vi "ManageRefs_FGV.vi"(7 "ManRef_mods":T1, 8 "error in":errorcluster, 11 "DataIn":variant) -> (0 "error out":errorcluster, 3 "DataOut":variant)   [LabVIEW 2017]
uses:
  ManRef_mods.ctl
  ManRef_AsterData.ctl
  ManRef_ShootData.ctl
  Asteroid/Asteroid_data.ctl
  GameConfig/GameConfig_data.ctl
  Asteroid/Asteroid_states.ctl
  Spaceship/Shoot/Shoot_states.ctl
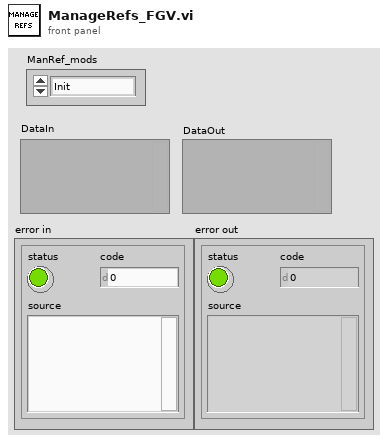
[diagram p1: front panel]
types:
  T1 = typedef "ManRef_mods.ctl" = enum16{"Init", "NewAster", "MoveAll", "DestroyAster", "NewShoot", "DestroyShot", "CheckColision", "End"}
  T2 = typedef "ManRef_ShootData.ctl" = cluster{"ID":i32, "ShootObjectRef":refnum<vi>}
  T3 = typedef "ManRef_AsterData.ctl" = cluster{"ID":i32, "AsterObjectRef":refnum<vi>}
  T4 = typedef "Asteroid_data.ctl" = cluster{"Veloc":dbl, "Direction":dbl, "Size":i32, "displayRef":refnum<vi>, "Max X":dbl, "Max Y":dbl, "Xpos":dbl, "Ypos":dbl, "ID":i32, "Config":T5}
  T5 = typedef "GameConfig_data.ctl" = cluster{"SpaceShip":cluster{"Angle":dbl, "SideLenght":dbl, "MaxLinearVeloc":dbl, "MaxAngularVeloc":dbl, "LinearAceleration":dbl, "AngularAceleration":dbl}, "Physics":cluster{"LinearDragFactor":dbl, "AngularDragFactor":dbl}, "Asteroids":cluster{"MaxSize":dbl, "MaxDivisions":i32, "MaxVeloc":dbl, "MinVeloc":dbl, "Fill":bool}, "Environment":cluster{"MaxAsteroids":i32, "TimeIncrement":dbl, "AsterProbCreation":dbl, "LogEnabled":bool}, "Shots":cluster{"MinTimeShots":dbl, "ShotSize":dbl, "ShotSpeed":dbl}}
  T6 = typedef "Shoot_states.ctl" = enum16{"Init", "Move", "Draw", "Destroy"}
  T7 = typedef "Asteroid_states.ctl" = enum16{"Init", "Move", "Split", "Draw", "Destroy"}
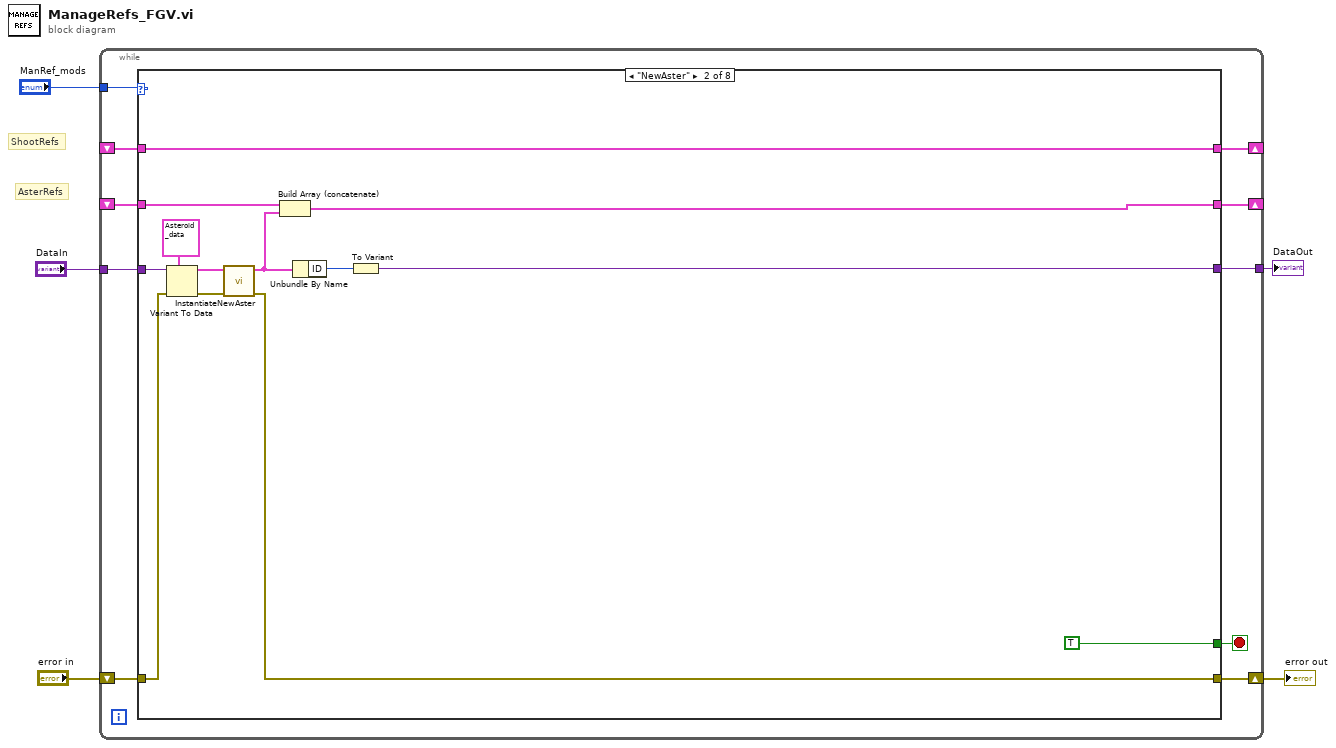
[diagram p0: block diagram]
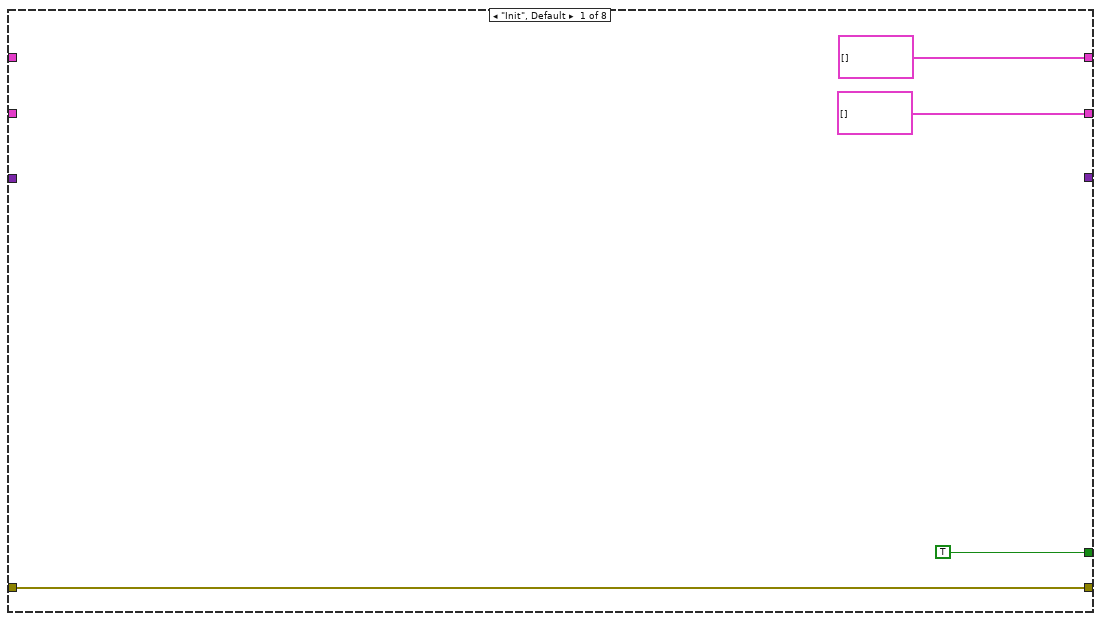
[diagram p2: hidden frame]
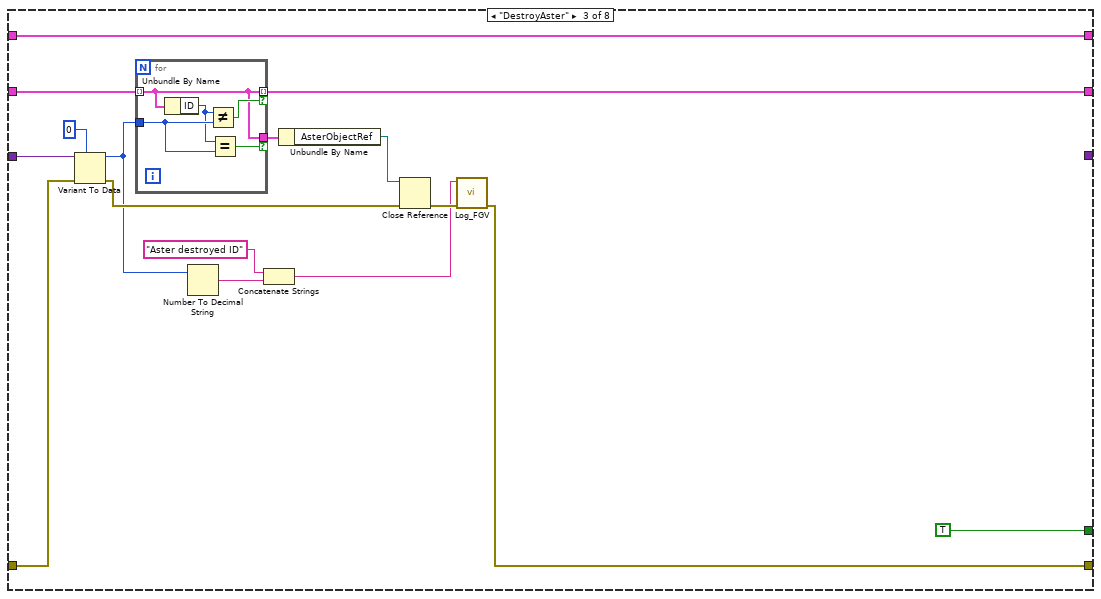
[diagram p3: hidden frame]
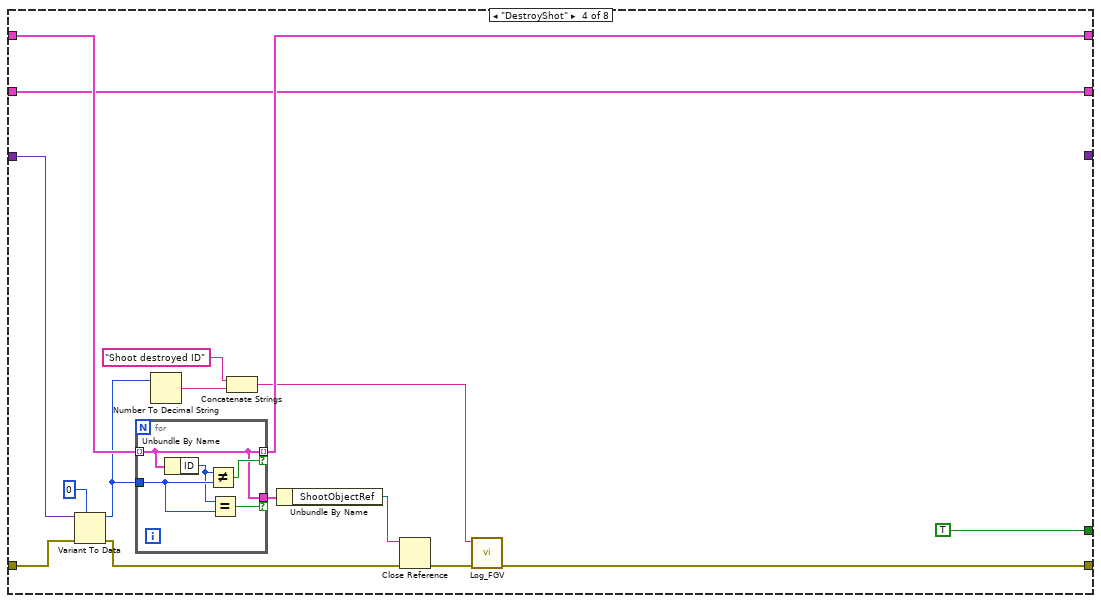
[diagram p4: hidden frame]
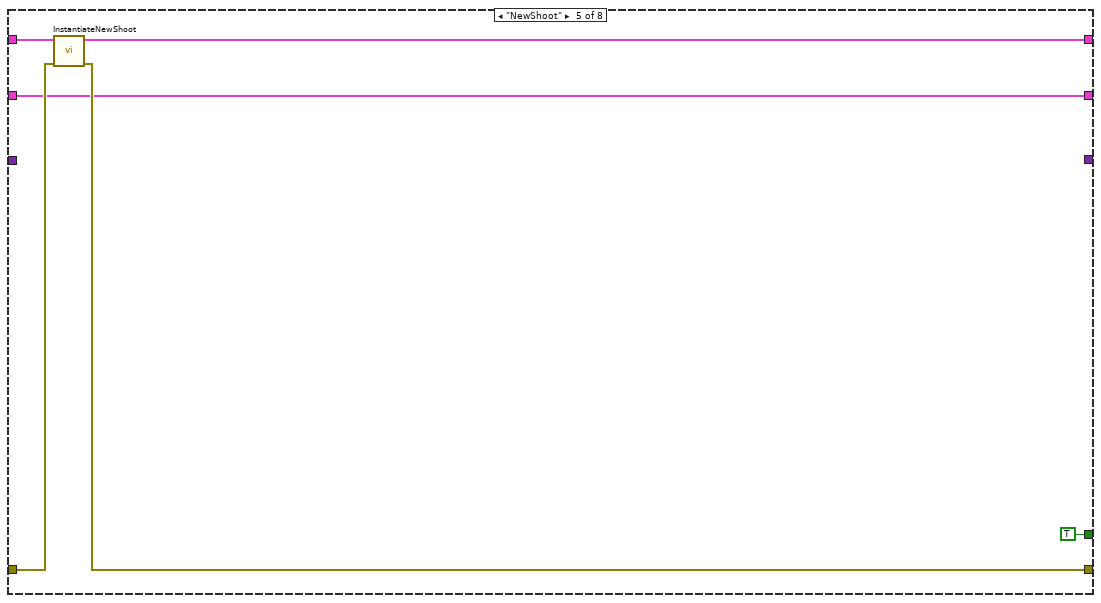
[diagram p5: hidden frame]
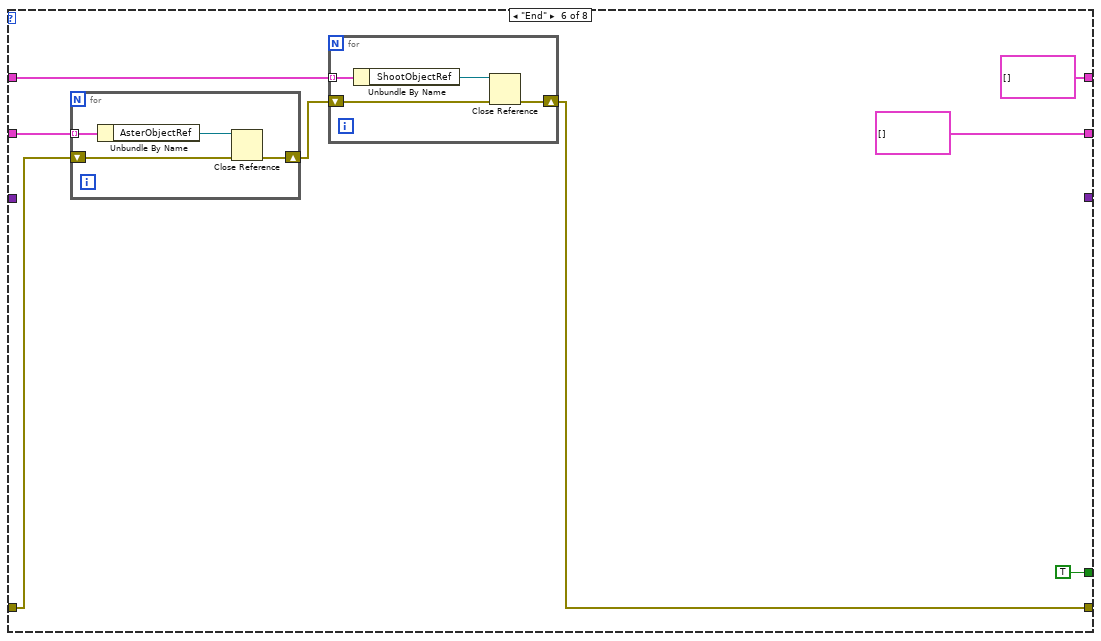
[diagram p6: hidden frame]
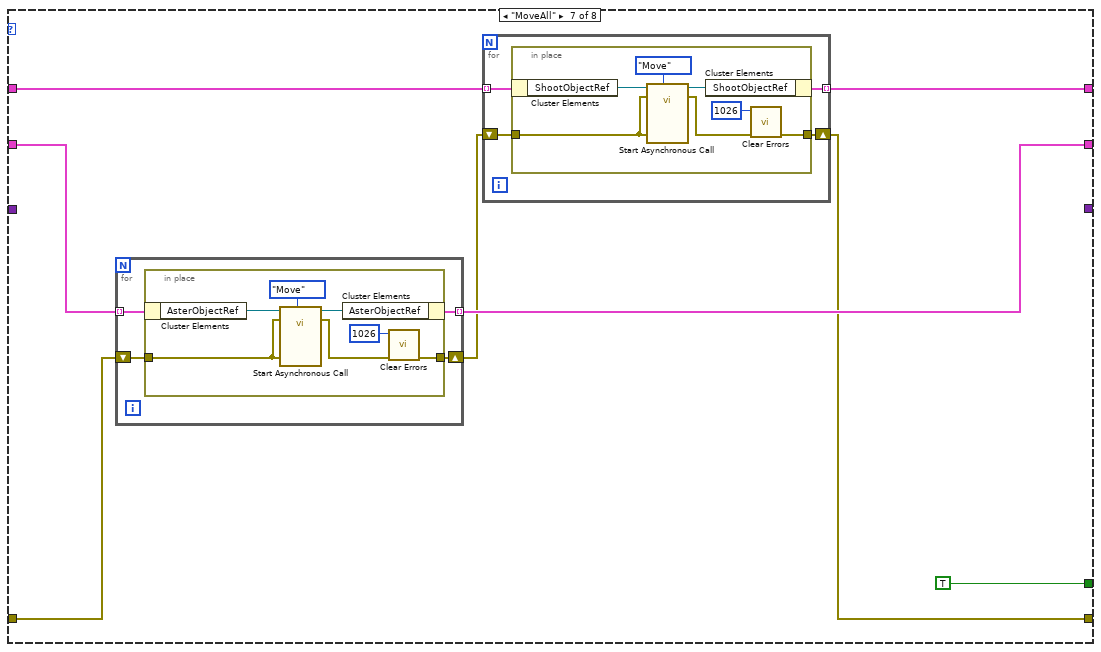
[diagram p7: hidden frame]
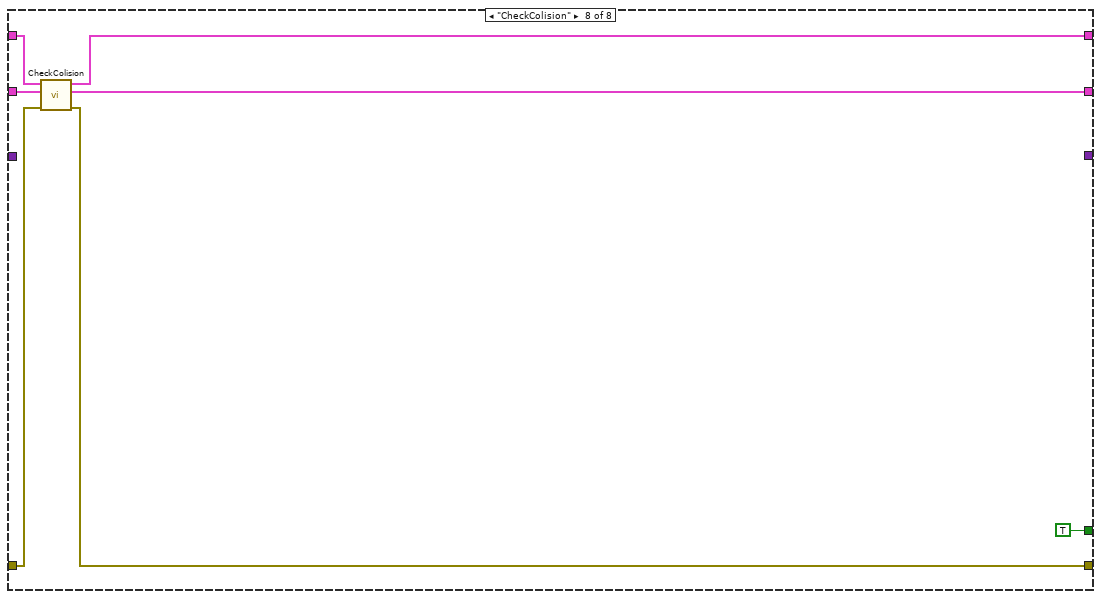
[diagram p8: hidden frame]
diagram:
  # "AsterRefs"
  # "ShootRefs"
  n1 = while {
    shift-right: [w12] -> w4
    shift-left: "error in" -> [w15]
    tunnel: "DataIn" -> [w14]
    tunnel: "ManRef_mods" -> [w13]
    shift-right: [w11] -> _
    shift-left: _ -> [w10]
    shift-right: [w8] -> _
    shift-left: _ -> [w7]
    tunnel: [w6] -> w1
    stop <- w9 stop-if-true
    n2 = case shown="\"NewAster\"" w13 {
      tunnel: w15 -> [w19 w24 w47 w68 w80 w86 w103 w132]
      tunnel: w14 -> [_ w32 w48 w69 _ _ _ _]
      tunnel: [w19 w29 w33 w54 w78 w82 w97 w127] -> w12
      tunnel: [T3[] [] ("appended array") w27 w44 w60 w75 T3[] [] ("appended array") w102 w131] -> w11
      tunnel: w10 -> [_ w28 w45 w60 w75 w87 w104 w133]
      tunnel: [TRUE ("empty?") TRUE ("empty?") TRUE ("empty?") TRUE ("empty?") TRUE ("empty?") TRUE ("empty?") TRUE ("empty?") TRUE ("empty?")] -> w9
      tunnel: [T2[] [] ("Array") w25 w39 w61 w76 T2[] [] ("Array") w98 w128] -> w8
      tunnel: w7 -> [_ w25 w39 w62 w77 w84 w100 w129]
      tunnel: [_ w20 _ _ _ _ _ _] -> w6
      frame "Init", Default {
      }
      frame "NewAster" {
        n3 = Variant To Data(error in=w24, type=T4 {"Veloc"=0.0, "Direction"=0.0, "Size"=0, "displayRef"=refnum, "Max X"=0.0, "Max Y"=0.0, "Xpos"=0.0, "Ypos"=0.0, "ID"=0, "Config"={"SpaceShip"={"Angle"=30.0, "SideLenght"=2.0, "MaxLinearVeloc"=10.0, "MaxAngularVeloc"=10.0, "LinearAceleration"=1.0, "AngularAceleration"=1.0}, "Physics"={"LinearDragFactor"=1.0, "AngularDragFactor"=1.0}, "Asteroids"={"MaxSize"=6.0, "MaxDivisions"=3, "MaxVeloc"=8.0, "MinVeloc"=1.0, "Fill"=FALSE}, "Environment"={"MaxAsteroids"=10, "TimeIncrement"=0.1, "AsterProbCreation"=0.1, "LogEnabled"=FALSE}, "Shots"={"MinTimeShots"=10.0, "ShotSize"=0.1, "ShotSpeed"=0.1}}} ("AsteroidData"), Variant=w32) -> (data=w30:T4, error out=w23:errorcluster)
        n4 = call "InstantiateNewAster.vi"("error in"=w23, "BaseAsteroidData"=w30) -> ("error out"=w29:errorcluster, "AsterRef"=w22:T3)  [unwired: 8 in]
        n5 = Build Array (concatenate)(w28, w22) -> (w27:T3[])
        n6 = Unbundle By Name(w22) -> ("ID"=w21:i32)
        n7 = To Variant(anything=w21) -> (Variant=w20:variant)
      }
      frame "DestroyAster" {
        n8 = Variant To Data(error in=w47, type=0, Variant=w48) -> (data=w36:i32, error out=w40:errorcluster)
        n9 = for {
          tunnel: w45 -> [w50] mode=indexing
          tunnel: w36 -> [w52]
          tunnel: [w50] -> w44 mode=indexing if=w53
          tunnel: [w50] -> w43 if=w49
          n10 = Unbundle By Name(w50) -> ("ID"=w51:i32)
          n11 = Not Equal?(x=w51, y=w52) -> (x != y?=w53:bool)
          n12 = Equal?(x=w51, y=w52) -> (x = y?=w49:bool)
        }
        n13 = Number To Decimal String(number=w36) -> (decimal integer string=w38:string)  [unwired: 1 in]
        n14 = Concatenate Strings("Aster destroyed ID" ("string"), w38) -> (w34:string)
        n15 = Unbundle By Name(w43) -> ("AsterObjectRef"=w41:refnum<vi>)
        n16 = Close Reference(reference=w41, error in (no error)=w40) -> (error out=w35:errorcluster)
        n17 = call "Log_FGV.vi"("error in"=w35, "Log"=w34) -> ("error out"=w33:errorcluster)  [unwired: 9 in]
      }
      frame "DestroyShot" {
        n18 = Variant To Data(error in=w68, type=0, Variant=w69) -> (data=w58:i32, error out=w63:errorcluster)
        n19 = for {
          tunnel: w62 -> [w71] mode=indexing
          tunnel: w58 -> [w73]
          tunnel: [w71] -> w61 mode=indexing if=w74
          tunnel: [w71] -> w66 if=w70
          n20 = Unbundle By Name(w71) -> ("ID"=w72:i32)
          n21 = Not Equal?(x=w72, y=w73) -> (x != y?=w74:bool)
          n22 = Equal?(x=w72, y=w73) -> (x = y?=w70:bool)
        }
        n23 = Number To Decimal String(number=w58) -> (decimal integer string=w57:string)  [unwired: 1 in]
        n24 = Concatenate Strings("Shoot destroyed ID" ("string"), w57) -> (w55:string)
        n25 = Unbundle By Name(w66) -> ("ShootObjectRef"=w64:refnum<vi>)
        n26 = Close Reference(reference=w64, error in (no error)=w63) -> (error out=w59:errorcluster)
        n27 = call "Log_FGV.vi"("error in"=w59, "Log"=w55) -> ("error out"=w54:errorcluster)  [unwired: 9 in]
      }
      frame "NewShoot" {
        n28 = call "InstantiateNewShoot.vi"("error in"=w80, "ShootsRef in"=w77) -> ("error out"=w78:errorcluster, "ShootsRef out"=w76:T2[])  [unwired: 8 in]
      }
      frame "End" {
        n29 = for {
          tunnel: w87 -> [w96] mode=indexing
          shift-right: [w93] -> w83
          shift-left: w86 -> [w94]
          n30 = Unbundle By Name(w96) -> ("AsterObjectRef"=w95:refnum<vi>)
          n31 = Close Reference(reference=w95, error in (no error)=w94) -> (error out=w93:errorcluster)
        }
        n32 = for {
          tunnel: w84 -> [w92] mode=indexing
          shift-right: [w89] -> w82
          shift-left: w83 -> [w90]
          n33 = Unbundle By Name(w92) -> ("ShootObjectRef"=w91:refnum<vi>)
          n34 = Close Reference(reference=w91, error in (no error)=w90) -> (error out=w89:errorcluster)
        }
      }
      frame "MoveAll" {
        n35 = for {
          tunnel: w104 -> [w119] mode=indexing
          shift-right: [w117] -> w99
          shift-left: w103 -> [w118]
          tunnel: [w116] -> w102 mode=indexing
          n36 = in-place {
            in-place-border: w118 -> [w125]
            in-place-border: [w120] -> w117
            n37 = in-place-cluster #1(w119) -> ("AsterObjectRef"=w126:refnum<vi>)
            n38 = call-by-ref "Start Asynchronous Call"(reference=w126, error in=w125, "Asteroid_states"=Asteroid_states."Move", "error in"=w125) -> (reference out=w124:refnum<vi>, error out=w121:errorcluster)  [unwired: 9 in, 1 out]
            n39 = in-place-cluster #1("AsterObjectRef"=w124) -> (w116:T3)
            n40 = call <vilib>:"Clear Errors.vi"("error in (no error)"=w121, "specific error code to clear (0: all)"=1026) -> ("error out"=w120:errorcluster)  [unwired: 4 in, 1 out]
          }
        }
        n41 = for {
          tunnel: w100 -> [w108] mode=indexing
          shift-right: [w106] -> w97
          shift-left: w99 -> [w107]
          tunnel: [w105] -> w98 mode=indexing
          n42 = in-place {
            in-place-border: w107 -> [w114]
            in-place-border: [w109] -> w106
            n43 = in-place-cluster #2(w108) -> ("ShootObjectRef"=w115:refnum<vi>)
            n44 = call-by-ref "Start Asynchronous Call"(reference=w115, error in=w114, "Shoot_states"=Shoot_states."Move", "error in"=w114) -> (reference out=w113:refnum<vi>, error out=w110:errorcluster)  [unwired: 9 in, 1 out]
            n45 = in-place-cluster #2("ShootObjectRef"=w113) -> (w105:T2)
            n46 = call <vilib>:"Clear Errors.vi"("error in (no error)"=w110, "specific error code to clear (0: all)"=1026) -> ("error out"=w109:errorcluster)  [unwired: 4 in, 1 out]
          }
        }
      }
      frame "CheckColision" {
        n47 = call "CheckColision.vi"("error in"=w132, "AsterRefs"=w133, "ShootsRef"=w129) -> ("error out"=w127:errorcluster, "AsterRefs out"=w131:T3[], "ShootsRef out"=w128:T2[])  [unwired: 6 in]
      }
    }
  }
  "error out" <- w4
  "DataOut" <- w1
